vi "xcorr bkp funciona MUX.vi"(4 "shift":u8, 5 "Pulse Energy":fxp<+,32,0>=0.99609375, 6 "N":u8, 7 "y":u32, 8 "x":u32, 9 "enable":bool, 10 "lag":u16) -> (1 "Rxy valid":bool, 2 "Rxy":u64, 3 "trigger":bool)   [LabVIEW 2017]
uses:
  <vilib>/rvi/FXPMathLib/basic elements/FxpDiscreteDelay/XNode/nifxpmath_DiscreteDelay.xnode
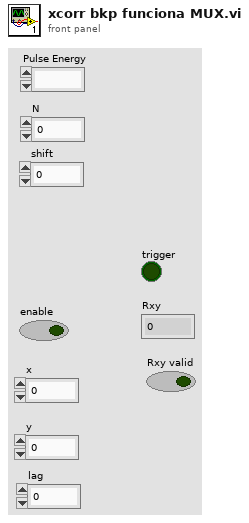
[diagram p1: front panel]
types:
  T1 = cluster{"Q":bool, "Q":bool, "Q":bool, "Q":bool, "Q":bool, "Q":bool, "Q":bool, "Q":bool, "Q":bool, "Q":bool, "Q":bool, "Q":bool, "Q":bool}
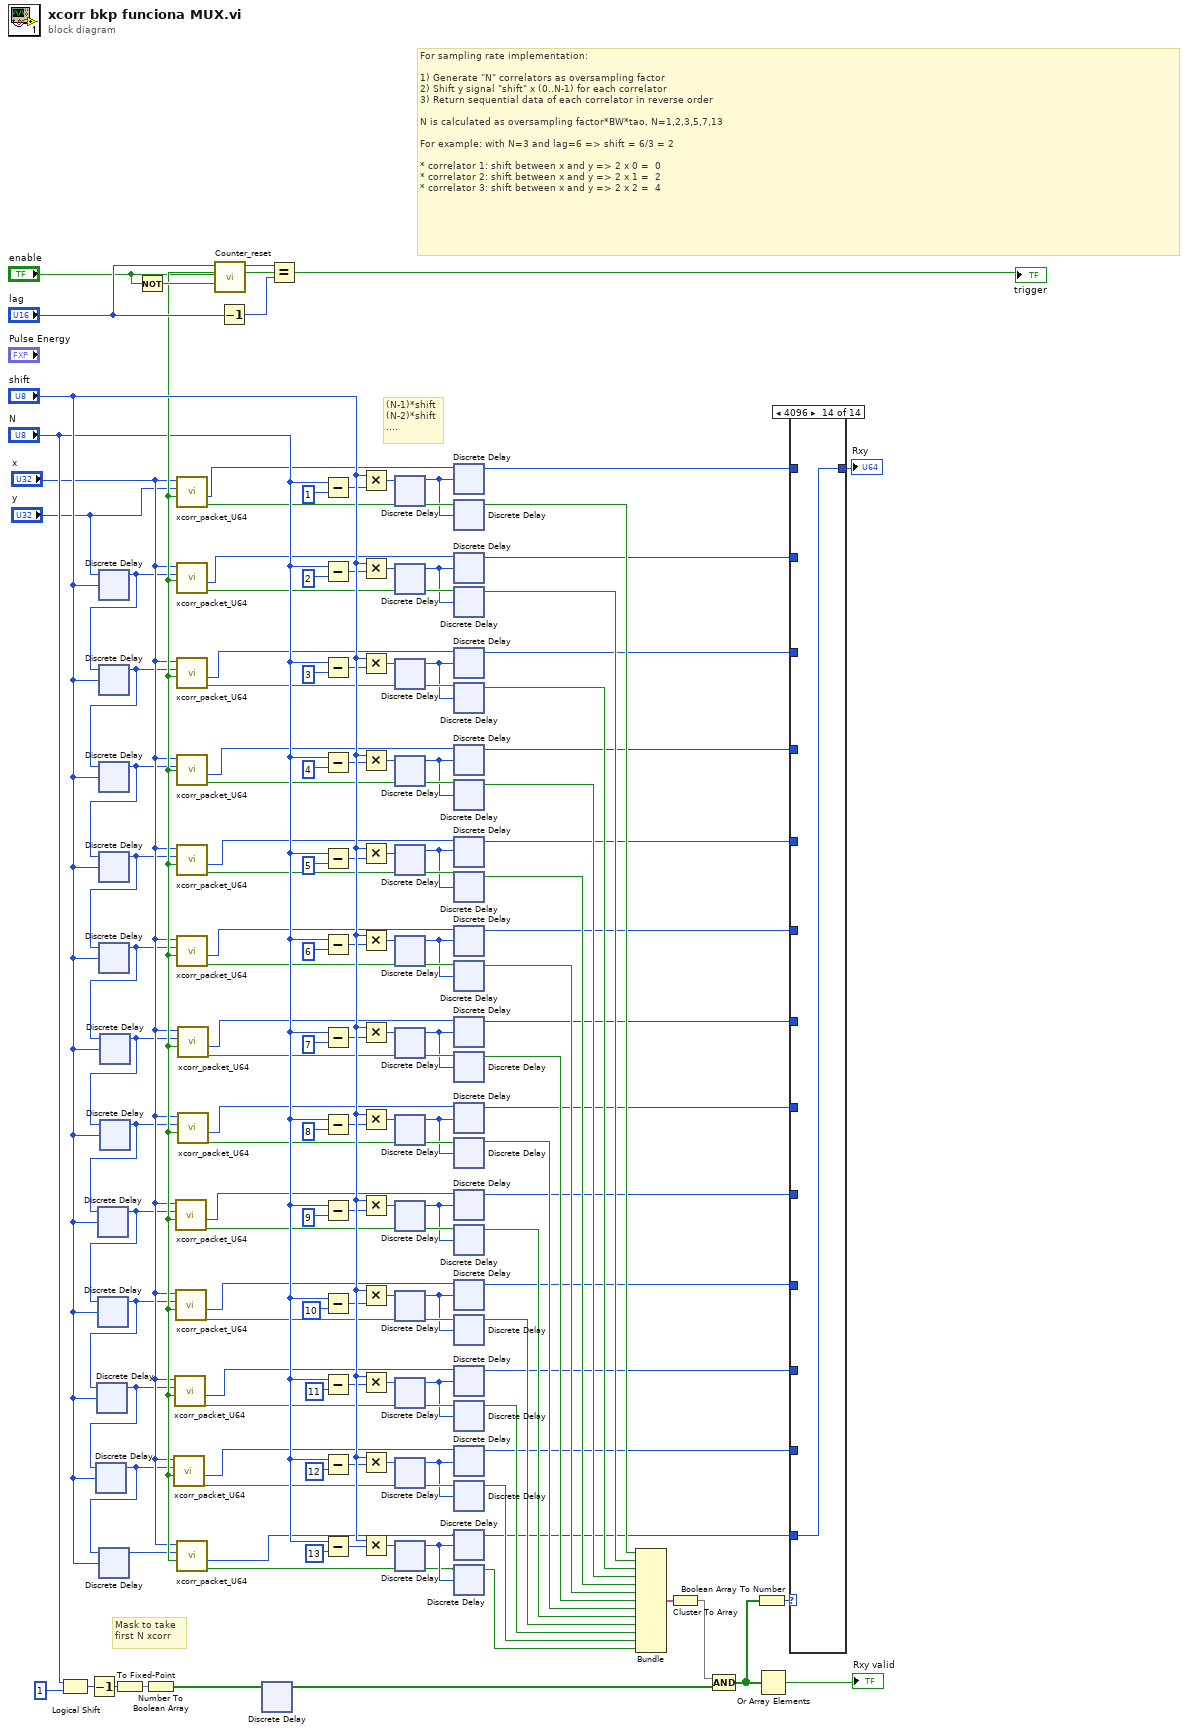
[diagram p0: block diagram]
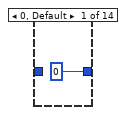
[diagram p2: hidden frame]
diagram:
  # "(N-1)*shift\n(N-2)*shift\n...."
  # "Mask to take \nfirst N xcorr"
  # "For sampling rate implementation:\n\n1) Generate \"N\" correlators as oversampling factor\n2) Shift y signal \"shift\" x (0..N-1) for each correlator\n3) Return sequential data of each correlator in reverse order\n\nN is calculated as oversampling factor*BW*tao, N=1,2,3,5,7,13\n\nFor example: with N=3 and lag=6 => shift = 6/3 = 2\n\n* correlator 1: shift between x and y => 2 x 0 =  0\n* correlator 2: shift between x and y => 2 x 1 =  2\n* correlator 3: shift between x and y => 2 x 2 =  4"
  n1 = Logical Shift(y="N", x=u16 1) -> (x << y=w130:u16)
  n2 = Decrement(x=w130) -> (x-1=w129:u16)
  n3 = xnode ("Discrete Delay")("D"="y", "n-1[0..255]"="shift") -> ("Q"=w76:u32)
  n4 = xnode ("Discrete Delay")("D"=w76, "n-1[0..255]"="shift") -> ("Q"=w86:u32)
  n5 = xnode ("Discrete Delay")("D"=w86, "n-1[0..255]"="shift") -> ("Q"=w85:u32)
  n6 = xnode ("Discrete Delay")("D"=w85, "n-1[0..255]"="shift") -> ("Q"=w84:u32)
  n7 = xnode ("Discrete Delay")("D"=w84, "n-1[0..255]"="shift") -> ("Q"=w83:u32)
  n8 = xnode ("Discrete Delay")("D"=w83, "n-1[0..255]"="shift") -> ("Q"=w82:u32)
  n9 = xnode ("Discrete Delay")("D"=w82, "n-1[0..255]"="shift") -> ("Q"=w81:u32)
  n10 = xnode ("Discrete Delay")("D"=w81, "n-1[0..255]"="shift") -> ("Q"=w80:u32)
  n11 = xnode ("Discrete Delay")("D"=w80, "n-1[0..255]"="shift") -> ("Q"=w79:u32)
  n12 = xnode ("Discrete Delay")("D"=w79, "n-1[0..255]"="shift") -> ("Q"=w78:u32)
  n13 = xnode ("Discrete Delay")("D"=w78, "n-1[0..255]"="shift") -> ("Q"=w77:u32)
  n14 = xnode ("Discrete Delay")("D"=w77, "n-1[0..255]"="shift") -> ("Q"=w108:u32)
  n15 = To Fixed-Point(number=w129) -> (fixed-point=w128:fxp<+,13,13>)  [unwired: 1 in]
  n16 = Not(x="enable") -> (.not. x?=w137:bool)
  n17 = Number To Boolean Array(number=w128) -> (Boolean array=w126:bool[])
  n18 = call "Counter_reset.vi"("reset"=w137, "enable"="enable", "limit"="lag") -> ("count"=w138:u16)  [unwired: 7 in, 1 out]
  n19 = Decrement(x="lag") -> (x-1=w135:u16)
  n20 = xnode ("Discrete Delay")("D"=w126) -> ("Q"=w18:bool[])
  n21 = Equal?(x=w138, y=w135) -> (x = y?=w133:bool)
  "trigger" <- w133
  n22 = call "xcorr_packet_U64.vi"("x"="x", "y"=w77, "trigger"=w133) -> ("out"=w87:u64, "valid"=w91:bool)  [unwired: 5 in]
  n23 = call "xcorr_packet_U64.vi"("x"="x", "y"=w78, "trigger"=w133) -> ("out"=w88:u64, "valid"=w96:bool)  [unwired: 5 in]
  n24 = call "xcorr_packet_U64.vi"("x"="x", "y"=w80, "trigger"=w133) -> ("out"=w99:u64, "valid"=w98:bool)  [unwired: 5 in]
  n25 = call "xcorr_packet_U64.vi"("x"="x", "y"=w79, "trigger"=w133) -> ("out"=w89:u64, "valid"=w97:bool)  [unwired: 5 in]
  n26 = call "xcorr_packet_U64.vi"("x"="x", "y"="y", "trigger"=w133) -> ("out"=w123:u64, "valid"=w122:bool)  [unwired: 5 in]
  n27 = call "xcorr_packet_U64.vi"("x"="x", "y"=w76, "trigger"=w133) -> ("out"=w114:u64, "valid"=w119:bool)  [unwired: 5 in]
  n28 = call "xcorr_packet_U64.vi"("x"="x", "y"=w86, "trigger"=w133) -> ("out"=w113:u64, "valid"=w118:bool)  [unwired: 5 in]
  n29 = call "xcorr_packet_U64.vi"("x"="x", "y"=w85, "trigger"=w133) -> ("out"=w112:u64, "valid"=w116:bool)  [unwired: 5 in]
  n30 = call "xcorr_packet_U64.vi"("x"="x", "y"=w84, "trigger"=w133) -> ("out"=w109:u64, "valid"=w107:bool)  [unwired: 5 in]
  n31 = call "xcorr_packet_U64.vi"("x"="x", "y"=w83, "trigger"=w133) -> ("out"=w110:u64, "valid"=w111:bool)  [unwired: 5 in]
  n32 = call "xcorr_packet_U64.vi"("x"="x", "y"=w108, "trigger"=w133) -> ("out"=w24:u64, "valid"=w23:bool)  [unwired: 5 in]
  n33 = call "xcorr_packet_U64.vi"("x"="x", "y"=w82, "trigger"=w133) -> ("out"=w105:u64, "valid"=w104:bool)  [unwired: 5 in]
  n34 = call "xcorr_packet_U64.vi"("x"="x", "y"=w81, "trigger"=w133) -> ("out"=w100:u64, "valid"=w101:bool)  [unwired: 5 in]
  n35 = Subtract(x="N", y=u8 1 ("x")) -> (x-y=w73:u8)
  n36 = Subtract(x="N", y=u8 2 ("x")) -> (x-y=w71:u8)
  n37 = Subtract(x="N", y=u8 3 ("x")) -> (x-y=w69:u8)
  n38 = Subtract(x="N", y=u8 4 ("x")) -> (x-y=w67:u8)
  n39 = Subtract(x="N", y=u8 5 ("x")) -> (x-y=w65:u8)
  n40 = Subtract(x="N", y=u8 6 ("x")) -> (x-y=w63:u8)
  n41 = Subtract(x="N", y=u8 7 ("x")) -> (x-y=w61:u8)
  n42 = Subtract(x="N", y=u8 8 ("x")) -> (x-y=w59:u8)
  n43 = Subtract(x="N", y=u8 9 ("x")) -> (x-y=w57:u8)
  n44 = Subtract(x="N", y=u8 10 ("x")) -> (x-y=w55:u8)
  n45 = Subtract(x="N", y=u8 11 ("x")) -> (x-y=w53:u8)
  n46 = Subtract(x="N", y=u8 12 ("x")) -> (x-y=w52:u8)
  n47 = Subtract(x="N", y=u8 13 ("x")) -> (x-y=w49:u8)
  n48 = Multiply(x="shift", y=w73) -> (x*y=w51:u8)
  n49 = Multiply(x="shift", y=w71) -> (x*y=w48:u8)
  n50 = Multiply(x="shift", y=w69) -> (x*y=w46:u8)
  n51 = Multiply(x="shift", y=w67) -> (x*y=w44:u8)
  n52 = Multiply(x="shift", y=w65) -> (x*y=w42:u8)
  n53 = Multiply(x="shift", y=w63) -> (x*y=w40:u8)
  n54 = Multiply(x="shift", y=w61) -> (x*y=w38:u8)
  n55 = Multiply(x="shift", y=w59) -> (x*y=w36:u8)
  n56 = Multiply(x="shift", y=w57) -> (x*y=w34:u8)
  n57 = Multiply(x="shift", y=w55) -> (x*y=w32:u8)
  n58 = Multiply(x="shift", y=w53) -> (x*y=w30:u8)
  n59 = Multiply(x="shift", y=w52) -> (x*y=w28:u8)
  n60 = Multiply(x="shift", y=w49) -> (x*y=w26:u8)
  n61 = xnode ("Discrete Delay")("D"=w51) -> ("Q"=w50:u8)
  n62 = xnode ("Discrete Delay")("D"=w48) -> ("Q"=w47:u8)
  n63 = xnode ("Discrete Delay")("D"=w46) -> ("Q"=w45:u8)
  n64 = xnode ("Discrete Delay")("D"=w44) -> ("Q"=w43:u8)
  n65 = xnode ("Discrete Delay")("D"=w42) -> ("Q"=w41:u8)
  n66 = xnode ("Discrete Delay")("D"=w40) -> ("Q"=w39:u8)
  n67 = xnode ("Discrete Delay")("D"=w38) -> ("Q"=w37:u8)
  n68 = xnode ("Discrete Delay")("D"=w36) -> ("Q"=w35:u8)
  n69 = xnode ("Discrete Delay")("D"=w34) -> ("Q"=w33:u8)
  n70 = xnode ("Discrete Delay")("D"=w32) -> ("Q"=w31:u8)
  n71 = xnode ("Discrete Delay")("D"=w30) -> ("Q"=w29:u8)
  n72 = xnode ("Discrete Delay")("D"=w28) -> ("Q"=w27:u8)
  n73 = xnode ("Discrete Delay")("D"=w26) -> ("Q"=w25:u8)
  n74 = xnode ("Discrete Delay")("D"=w123, "n-1[0..255]"=w50) -> ("Q"=w15:u64)
  n75 = xnode ("Discrete Delay")("D"=w122, "n-1[0..255]"=w50) -> ("Q"=w121:bool)
  n76 = xnode ("Discrete Delay")("D"=w114, "n-1[0..255]"=w47) -> ("Q"=w14:u64)
  n77 = xnode ("Discrete Delay")("D"=w119, "n-1[0..255]"=w47) -> ("Q"=w120:bool)
  n78 = xnode ("Discrete Delay")("D"=w113, "n-1[0..255]"=w45) -> ("Q"=w13:u64)
  n79 = xnode ("Discrete Delay")("D"=w118, "n-1[0..255]"=w45) -> ("Q"=w117:bool)
  n80 = xnode ("Discrete Delay")("D"=w112, "n-1[0..255]"=w43) -> ("Q"=w12:u64)
  n81 = xnode ("Discrete Delay")("D"=w116, "n-1[0..255]"=w43) -> ("Q"=w115:bool)
  n82 = xnode ("Discrete Delay")("D"=w109, "n-1[0..255]"=w41) -> ("Q"=w11:u64)
  n83 = xnode ("Discrete Delay")("D"=w107, "n-1[0..255]"=w41) -> ("Q"=w106:bool)
  n84 = xnode ("Discrete Delay")("D"=w110, "n-1[0..255]"=w39) -> ("Q"=w10:u64)
  n85 = xnode ("Discrete Delay")("D"=w111, "n-1[0..255]"=w39) -> ("Q"=w20:bool)
  n86 = xnode ("Discrete Delay")("D"=w105, "n-1[0..255]"=w37) -> ("Q"=w9:u64)
  n87 = xnode ("Discrete Delay")("D"=w104, "n-1[0..255]"=w37) -> ("Q"=w103:bool)
  n88 = xnode ("Discrete Delay")("D"=w100, "n-1[0..255]"=w35) -> ("Q"=w8:u64)
  n89 = xnode ("Discrete Delay")("D"=w101, "n-1[0..255]"=w35) -> ("Q"=w95:bool)
  n90 = xnode ("Discrete Delay")("D"=w99, "n-1[0..255]"=w33) -> ("Q"=w7:u64)
  n91 = xnode ("Discrete Delay")("D"=w98, "n-1[0..255]"=w33) -> ("Q"=w94:bool)
  n92 = xnode ("Discrete Delay")("D"=w89, "n-1[0..255]"=w31) -> ("Q"=w6:u64)
  n93 = xnode ("Discrete Delay")("D"=w97, "n-1[0..255]"=w31) -> ("Q"=w93:bool)
  n94 = xnode ("Discrete Delay")("D"=w88, "n-1[0..255]"=w29) -> ("Q"=w5:u64)
  n95 = xnode ("Discrete Delay")("D"=w96, "n-1[0..255]"=w29) -> ("Q"=w92:bool)
  n96 = xnode ("Discrete Delay")("D"=w87, "n-1[0..255]"=w27) -> ("Q"=w4:u64)
  n97 = xnode ("Discrete Delay")("D"=w91, "n-1[0..255]"=w27) -> ("Q"=w90:bool)
  n98 = xnode ("Discrete Delay")("D"=w24, "n-1[0..255]"=w25) -> ("Q"=w3:u64)
  n99 = xnode ("Discrete Delay")("D"=w23, "n-1[0..255]"=w25) -> ("Q"=w22:bool)
  n100 = Bundle("Q"=w121, "Q"=w120, "Q"=w117, "Q"=w115, "Q"=w106, "Q"=w20, "Q"=w103, "Q"=w95, "Q"=w94, "Q"=w93, "Q"=w92, "Q"=w90, "Q"=w22) -> (w102:T1)  [unwired: 1 in]
  n101 = Cluster To Array(cluster=w102) -> (array=w75:bool[])
  n102 = Compound Arithmetic op=AND(w75, w18) -> (w16:bool[])
  n103 = Boolean Array To Number(Boolean array=w16) -> (number=w21:u16)
  n104 = Or Array Elements(Boolean array=w16) -> (logical OR=→"Rxy valid":bool)
  n105 = case shown="4096" w21 {
    tunnel: [u64 0 ("out") w140 w141 w142 w143 w144 w145 w146 w147 w148 w149 w150 w151 w152] -> w2
    tunnel: w15 -> [_ w140 _ _ _ _ _ _ _ _ _ _ _ _]
    tunnel: w14 -> [_ _ w141 _ _ _ _ _ _ _ _ _ _ _]
    tunnel: w13 -> [_ _ _ w142 _ _ _ _ _ _ _ _ _ _]
    tunnel: w12 -> [_ _ _ _ w143 _ _ _ _ _ _ _ _ _]
    tunnel: w11 -> [_ _ _ _ _ w144 _ _ _ _ _ _ _ _]
    tunnel: w10 -> [_ _ _ _ _ _ w145 _ _ _ _ _ _ _]
    tunnel: w3 -> [_ _ _ _ _ _ _ _ _ _ _ _ _ w152]
    tunnel: w9 -> [_ _ _ _ _ _ _ w146 _ _ _ _ _ _]
    tunnel: w8 -> [_ _ _ _ _ _ _ _ w147 _ _ _ _ _]
    tunnel: w7 -> [_ _ _ _ _ _ _ _ _ w148 _ _ _ _]
    tunnel: w5 -> [_ _ _ _ _ _ _ _ _ _ _ w150 _ _]
    tunnel: w4 -> [_ _ _ _ _ _ _ _ _ _ _ _ w151 _]
    tunnel: w6 -> [_ _ _ _ _ _ _ _ _ _ w149 _ _ _]
    frame 0, Default {
    }
    frame 1 {
    }
    frame 2 {
    }
    frame 4 {
    }
    frame 8 {
    }
    frame 16 {
    }
    frame 32 {
    }
    frame 64 {
    }
    frame 128 {
    }
    frame 256 {
    }
    frame 512 {
    }
    frame 1024 {
    }
    frame 2048 {
    }
    frame 4096 {
    }
  }
  "Rxy" <- w2
